vi "Set Plug-in Name Warning.vi"(0 "Valid Name?":bool[](array[boolean]), 5 "Validated names":string[](array[string]), 11 "error in (no error)":errorcluster) -> (4 "Warning?":bool, 15 "error out":errorcluster)   [LabVIEW 2021, in "Migrator.lvlib"]
uses:
  Migrator.lvlib
  9493a277-5240-4c57-92b6-b8f5b809ca06.vi
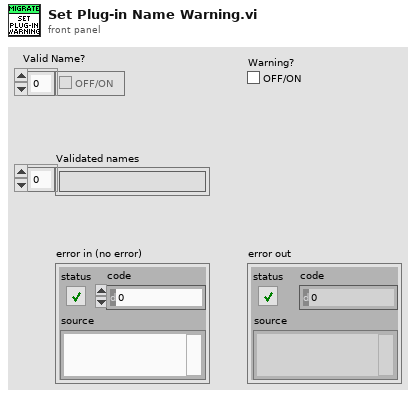
[diagram p1: front panel]
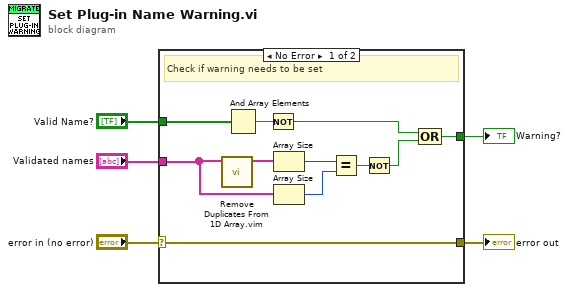
[diagram p0: block diagram]
diagram:
  n1 = case shown="No Error" "error in (no error)" {
    selector: "error in (no error)" -> [w16 w17]
    tunnel: [w15 _] -> w5
    tunnel: "Validated names" -> [w9 _]
    tunnel: [w16 w17] -> w2
    tunnel: "Valid Name?" -> [w8 _]
    frame No Error {
      # "Check if warning needs to be set"
      n2 = call "Remove Duplicates From 1D Array.vim"("array"=w9) -> ("array with duplicates removed"=w14:string[])  [unwired: 10 in]
      n3 = And Array Elements(Boolean array=w8) -> (logical AND=w7:bool)
      n4 = Not(x=w7) -> (.not. x?=w6:bool)
      n5 = Array Size(array=w14) -> (size(s)=w13:i32)
      n6 = Array Size(array=w9) -> (size(s)=w12:i32)
      n7 = Equal?(x=w13, y=w12) -> (x = y?=w11:bool)
      n8 = Not(x=w11) -> (.not. x?=w10:bool)
      n9 = Compound Arithmetic op=OR(w6, w10) -> (w15:bool)
    }
    frame Error {
      # "Pass"
    }
  }
  "Warning?" <- w5
  "error out" <- w2
